vi "DFT 64 (SubVI).vi"(10 "Datos":dbl[](array[numeric]), 11 "WaveformGraph in":refnum<vi>) -> (2 "DFT (N=64)":dbl[](graph), 3 "Array":dbl[](array[numeric]))   [LabVIEW 2020]
uses:
  <vilib>/Analysis/2dsp.llb/Real FFT.vi
  <vilib>/Analysis/NI_AALPro.lvlib
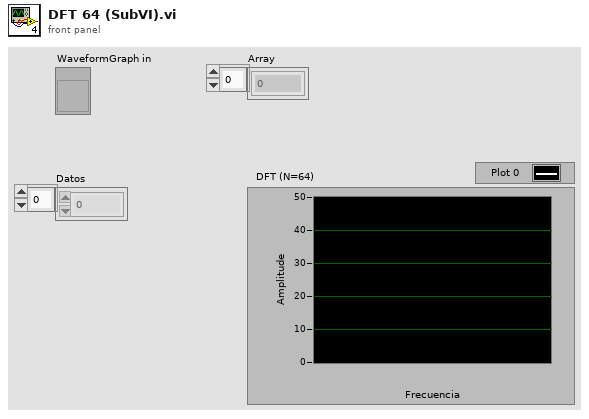
[diagram p1: front panel]
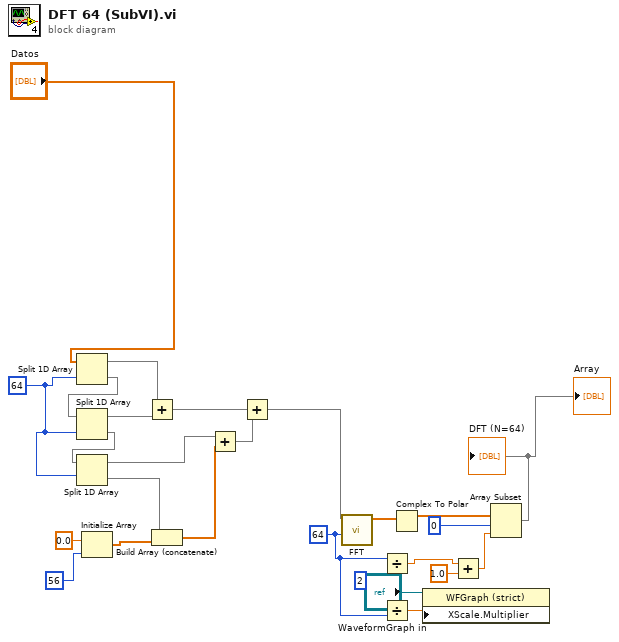
[diagram p0: block diagram]
diagram:
  w12 = 2 ("x")
  w13 = 64 ("FFT size")
  w5 = 64 ("index")
  n1 = Split 1D Array(array="Datos", index=w5) -> (first subarray=w18:dbl[], second subarray=w3:dbl[])
  n2 = Split 1D Array(array=w3, index=w5) -> (first subarray=w19:dbl[], second subarray=w4:dbl[])
  n3 = Split 1D Array(array=w4, index=w5) -> (first subarray=w21:dbl[], second subarray=w20:dbl[])
  n4 = Initialize Array(0.0 ("element"), 56 ("dimension size")) -> (w2:dbl[])
  n5 = Add(x=w18, y=w19) -> (x+y=w23:dbl[])
  n6 = Build Array (concatenate)(w20, w2) -> (w22:dbl[])
  n7 = Add(x=w21, y=w22) -> (x+y=w24:dbl[])
  n8 = Add(x=w23, y=w24) -> (x+y=w25:dbl[])
  n9 = call-poly <vilib>:"FFT.vi"("FFT size"=w13, "X"=w25) -> ("FFT {X}"=w6:cdb[])  [unwired: 8 in, 1 out]
  n10 = Divide(x=w13, y=w12) -> (x/y=w9:dbl)
  n11 = Divide(x=w12, y=w13) -> (x/y=w14:dbl)
  n12 = Complex To Polar(r * e^(i*theta)=w6) -> (r=w7:dbl[])  [unwired: 1 out]
  n13 = property on="Property Node" class="WFGraph (strict)"(reference="WaveformGraph in", "XScale.Multiplier"=w14) -> ()  [unwired: 1 in, 2 out]
  n14 = Add(x=w9, y=1.0) -> (x+y=w11:dbl)
  n15 = Array Subset(array=w7, index=0, length=w11) -> (→"DFT (N=64)" →"Array":dbl[])
